vi "pp_trialType_fromStringArray.vi"(8 "error in (no error)":errorcluster, 11 "Input string array":string[](array[string])=["1", "GO", "0", "FM Sweep", "2.000000", "4.000000", "0.000000"]) -> (0 "error out":errorcluster, 3 "Ouptut Trial Cluster":T1={"Trial Code"=0, "Trial Type"=enum."NOGO", "Trial Weight"=0, "Stim Type"=enum."Pure Tone", "Stim Dur (s)"=0.0, "Stim P1"=0.0, "Stim P2"=0.0} {"Stim P2" min=0.0; "Trial Weight" step=1; "Stim P1" min=0.0; "Stim Dur (s)" min=0.0; "Trial Code" min=1 step=1})   [LabVIEW 2013]
uses:
  labolabo/array/impl/ArrayRead_S.vi
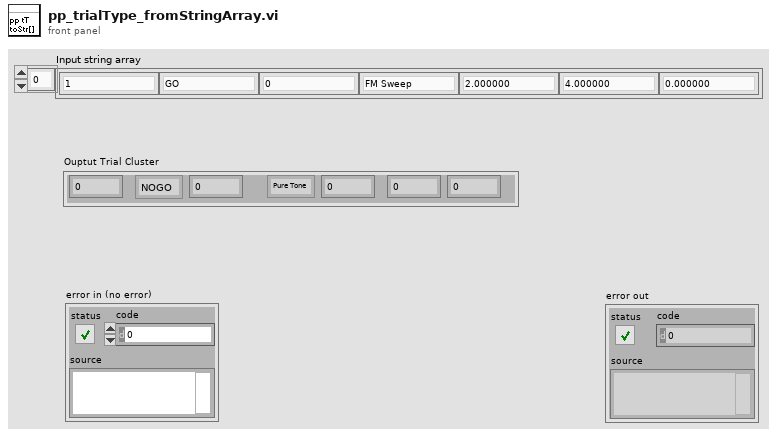
[diagram p1: front panel]
types:
  T1 = cluster{"Trial Code":u16, "Trial Type":enum16{"OFF", "GO", "NOGO", "TEST"}, "Trial Weight":u32, "Stim Type":enum16{"Pure Tone", "FM Sweep"}, "Stim Dur (s)":dbl, "Stim P1":dbl, "Stim P2":dbl}
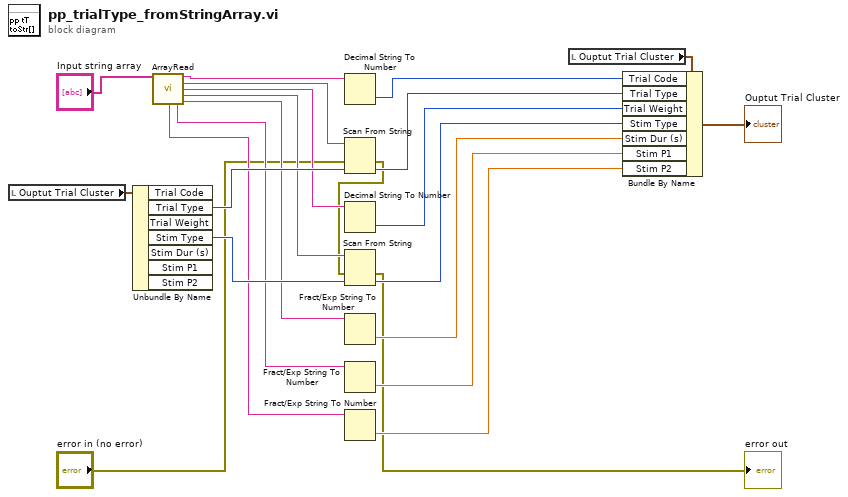
[diagram p0: block diagram]
diagram:
  n1 = local read "Ouptut Trial Cluster"() -> (w17:T1)
  n2 = Unbundle By Name(w17) -> ("Trial Type"=w16:enum16{"OFF", "GO", "NOGO", "TEST"}, "Stim Type"=w12:enum16{"Pure Tone", "FM Sweep"})  [unwired: 5 out]
  n3 = call-poly "ArrayRead.vi"("Current (or Cued Trial Parameters)"="Input string array") -> ("Value 0"=w20:string, "Value 1"=w18:string, "Value 2"=w14:string, "Value 3"=w11:string, "Value 6"=w5:string, "Value 5"=w7:string, "Value 4"=w9:string)  [unwired: 6 in, 2 out]
  n4 = Decimal String To Number(string=w20) -> (number=w19:i32)  [unwired: 2 in, 1 out]
  n5 = Scan From String(input string=w18, error in="error in (no error)", default 1=w16) -> (error out=w2:errorcluster, output 1=w15:enum16{"OFF", "GO", "NOGO", "TEST"})  [unwired: 2 in, 2 out]
  n6 = Decimal String To Number(string=w14) -> (number=w13:i32)  [unwired: 2 in, 1 out]
  n7 = Scan From String(input string=w11, error in=w2, default 1=w12) -> (error out=→"error out":errorcluster, output 1=w10:enum16{"Pure Tone", "FM Sweep"})  [unwired: 2 in, 2 out]
  n8 = Fract/Exp String To Number(string=w9) -> (number=w8:dbl)  [unwired: 3 in, 1 out]
  n9 = Fract/Exp String To Number(string=w7) -> (number=w6:dbl)  [unwired: 3 in, 1 out]
  n10 = Fract/Exp String To Number(string=w5) -> (number=w4:dbl)  [unwired: 3 in, 1 out]
  n11 = local read "Ouptut Trial Cluster"() -> (w23:T1)
  n12 = Bundle By Name(cluster=w23, "Trial Code"=w19, "Trial Type"=w15, "Trial Weight"=w13, "Stim Type"=w10, "Stim Dur (s)"=w8, "Stim P1"=w6, "Stim P2"=w4) -> (→"Ouptut Trial Cluster":T1)
